vi "unix_time_nanoseconds.vi"() -> (3 "String":string)   [LabVIEW 2018]
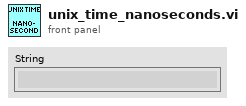
[diagram p1: front panel]
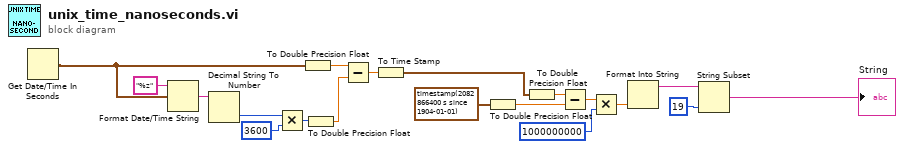
[diagram p0: block diagram]
diagram:
  n1 = Get Date/Time In Seconds() -> (seconds since 1Jan1904=w16:timestamp)
  n2 = Format Date/Time String(time format string (%c)="%z", seconds (now)=w16) -> (date/time string=w14:string)  [unwired: 1 out]
  n3 = Decimal String To Number(string=w14) -> (number=w15:i32)  [unwired: 3 out]
  n4 = Multiply(x=w15, y=3600) -> (x*y=w10:i32)
  n5 = To Double Precision Float(number=w16) -> (double precision float=w11:dbl)
  n6 = To Double Precision Float(number=w10) -> (double precision float=w12:dbl)
  n7 = Subtract(x=w11, y=w12) -> (x-y=w13:dbl)
  n8 = To Time Stamp(1:w13) -> (0:w17:timestamp)
  n9 = To Double Precision Float(number=timestamp(2082866400 s since 1904-01-01)) -> (double precision float=w7:dbl)
  n10 = To Double Precision Float(number=w17) -> (double precision float=w6:dbl)
  n11 = Subtract(x=w6, y=w7) -> (x-y=w18:dbl)
  n12 = Multiply(x=w18, y=1000000000) -> (x*y=w4:dbl)
  n13 = Format Into String(w4) -> (resulting string=w3:string)  [unwired: 3 in, 1 out]
  n14 = String Subset(string=w3, length (rest)=19) -> (substring=→"String":string)  [unwired: 1 in]
